vi "Add Viewer.vi"(8 "error in":errorcluster, 10 "viewer":T1, 11 "Data Server Thread in":refnum<class "Data Server Thread.lvclass">) -> (0 "error out":errorcluster, 3 "Data Server Thread out":refnum<class "Data Server Thread.lvclass">)   [LabVIEW 2020, in "DSF Core.lvlib" / "Data Server Thread.lvclass"]
uses:
  Data Server Thread.lvclass
  Viewer Data.ctl
  Buffer/Buffer.lvclass
  Status/Status Pointer.lvclass
  Data Server Thread.lvclass/Data Server Thread.ctl
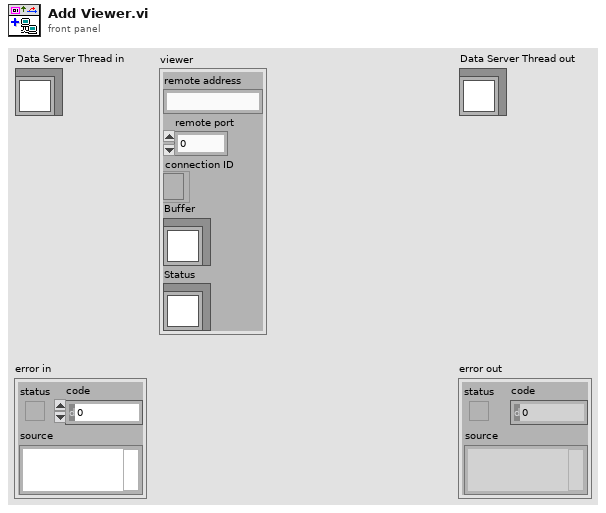
[diagram p1: front panel]
types:
  T1 = typedef "DSF Core.lvlib/Data Server Thread.lvclass/Viewer Data.ctl" = cluster{"remote address":string, "remote port":u16, "connection ID":refnum<k5>, "Buffer":refnum<class "Buffer.lvclass">, "Status":refnum<class "Status Pointer.lvclass">}
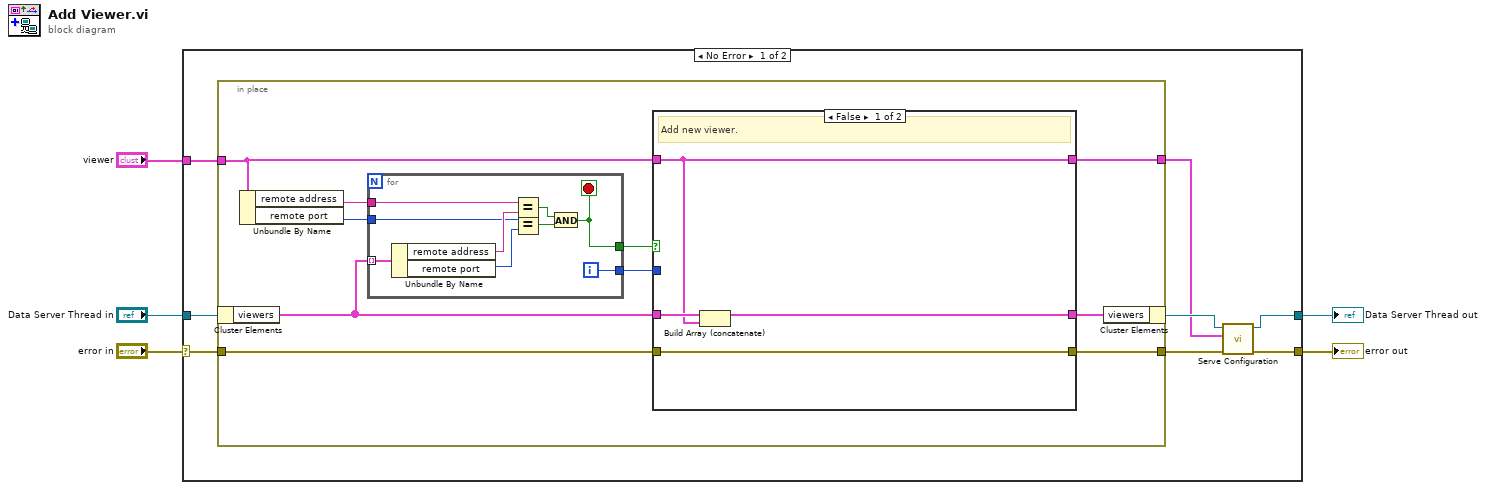
[diagram p0: block diagram]
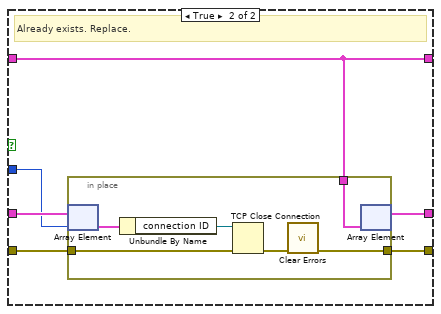
[diagram p2: hidden frame]
diagram:
  n1 = case shown="No Error" "error in" {
    selector: "error in" -> [w11 w50]
    tunnel: "Data Server Thread in" -> [w13 w49]
    tunnel: "viewer" -> [w12 _]
    tunnel: [w9 w50] -> w3
    tunnel: [w7 w49] -> w2
    frame No Error {
      n2 = in-place {
        in-place-border: w12 -> [w20]
        in-place-border: w11 -> [w18]
        in-place-border: [w17] -> w10
        in-place-border: [w16] -> w6
        n3 = in-place-cluster #1(w13) -> ("viewers"=w15:T1[])
        n4 = Unbundle By Name(w20) -> ("remote address"=w23:string, "remote port"=w14:u16)
        n5 = for {
          tunnel: w15 -> [w48] mode=indexing
          tunnel: w23 -> [w43]
          tunnel: [w40] -> w22
          tunnel: [w46] -> w19
          tunnel: w14 -> [w45]
          i -> [w46]
          stop <- w40 stop-if-true
          n6 = Unbundle By Name(w48) -> ("remote address"=w47:string, "remote port"=w44:u16)
          n7 = Equal?(x=w43, y=w47) -> (x = y?=w41:bool)
          n8 = Equal?(x=w45, y=w44) -> (x = y?=w42:bool)
          n9 = And(x=w41, y=w42) -> (x .and. y?=w40:bool)
        }
        n10 = case shown="False" w22 {
          tunnel: w15 -> [w26 w30]
          tunnel: [w27 w33] -> w21
          tunnel: w20 -> [w24 w28]
          tunnel: w19 -> [_ w29]
          tunnel: w18 -> [w25 w32]
          tunnel: [w25 w31] -> w17
          tunnel: [w24 w28] -> w16
          frame False {
            # "Add new viewer."
            n11 = Build Array (concatenate)(w26, w24) -> (w27:T1[])
          }
          frame True {
            # "Already exists. Replace."
            n12 = in-place {
              in-place-border: [w34] -> w31
              in-place-border: w28 -> [w37]
              in-place-border: w32 -> [w36]
              n13 = in-place-array #2(w30, w29) -> (w39:T1)
              n14 = Unbundle By Name(w39) -> ("connection ID"=w38:refnum<k5>)
              n15 = TCP Close Connection(connection ID=w38, error in (no error)=w36) -> (error out=w35:errorcluster)  [unwired: 1 in, 1 out]
              n16 = call <vilib>:"Clear Errors.vi"("error in (no error)"=w35) -> ("error out"=w34:errorcluster)  [unwired: 5 in, 1 out]
              n17 = in-place-array #2(w37) -> (w33:T1[])  [unwired: 1 out]
            }
          }
        }
        n18 = in-place-cluster #1("viewers"=w21) -> (w8:refnum<class "Data Server Thread.lvclass">)
      }
      n19 = call "Serve Configuration.vi"("error in"=w10, "viewer"=w6, "Data Server Thread in"=w8) -> ("error out"=w9:errorcluster, "Data Server Thread out"=w7:refnum<class "Data Server Thread.lvclass">)  [unwired: 7 in]
    }
    frame Error {
    }
  }
  "error out" <- w3
  "Data Server Thread out" <- w2
